vi "RSZVB Calibration Auto with Timeout.vi"(0 "VISA session":refnum<visa-resource-name>, 1 "Channel (1)":i32=1, 2 "Calibration Kit Name":string, 3 "Timeout (50000 ms)":i32=50000, 5 "error in (no error)":errorcluster {"code" format="%.0x"}, 6 "Analyzer Port 1 (1)":i32=1, 7 "Cal Unit Port 1 (1)":i32=1, 8 "Analyzer Port 2 (1)":i32=1, 9 "Cal Unit Port 2 (1)":i32=1, 10 "Analyzer Port 3 (1)":i32=1, 11 "Cal Unit Port 3 (1)":i32=1, 12 "Analyzer Port 4 (1)":i32=1, 13 "Cal Unit Port 4 (1)":i32=1) -> (14 "dup VISA session":refnum<visa-resource-name>, 19 "error out":errorcluster {"code" format="%.0x"})   [LabVIEW 2011]
doc: "This VI selects and initiates a one-port, two-port, three-port or four-port automatic calibration at arbitrary analyzer and calibration unit ports.\n\nNote(s):\n\n(1) Port numbers of the analyzer:\nFor an n-port automatic calibration (n = 1 to 4), n arbitrary (not necessarily consecutive) port numbers must be specified.\n\n(2) Port numbers of the cal unit:\nFor an n-port automatic calibration (n = 1 to 4), n arbitrary (not necessarily consecutive) port numbers must be specified. It is possible to combine arbitrary (not necessarily matching) pairs of analyzer and cal unit ports.\n \nRemote-control command(s):\n[SENSe<Ch>:]CORRection:COLLect:AUTO:PORTs '<file_name>',<analyzer_port_no>,<cal_unit_port_no>{,<analyzer_port_no>,<cal_unit_port_no>}"
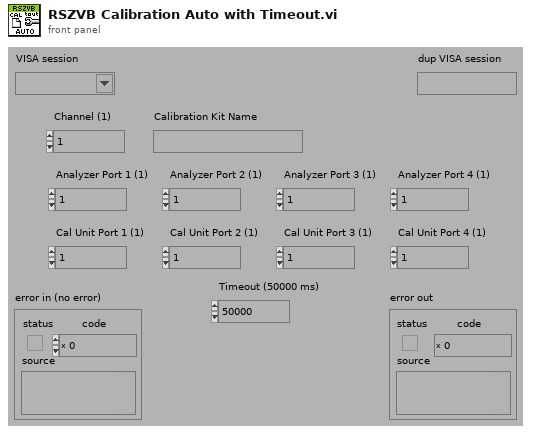
[diagram p1: front panel]
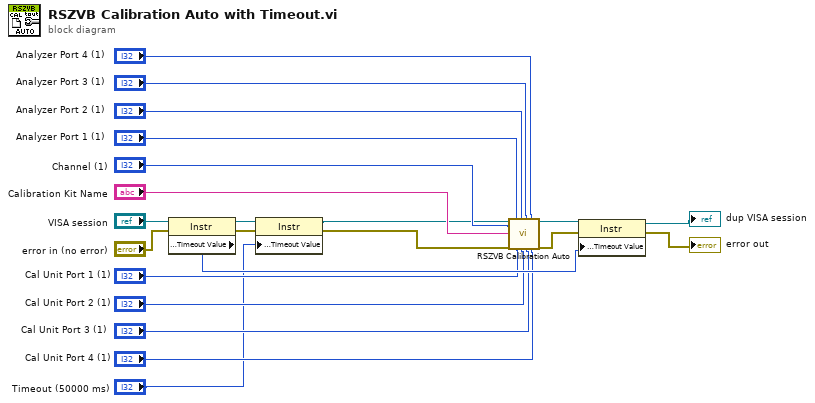
[diagram p0: block diagram]
diagram:
  n1 = property class="Instr"(reference="VISA session", error in="error in (no error)") -> (reference out=w5:refnum<visa-resource-name>, error out=w4:errorcluster, "General Settings:Timeout Value"=w20:u32)
  n2 = property class="Instr"(reference=w5, error in=w4, "General Settings:Timeout Value"="Timeout (50000 ms)") -> (reference out=w1:refnum<visa-resource-name>, error out=w2:errorcluster)
  n3 = call "RSZVB Calibration Auto.vi"("VISA session"=w1, "Channel (1)"="Channel (1)", "Calibration Kit Name"="Calibration Kit Name", "error in (no error)"=w2, "Analyzer Port 1 (1)"="Analyzer Port 1 (1)", "Cal Unit Port 1 (1)"="Cal Unit Port 1 (1)", "Analyzer Port 2 (1)"="Analyzer Port 2 (1)", "Cal Unit Port 2 (1)"="Cal Unit Port 2 (1)", "Analyzer Port 3 (1)"="Analyzer Port 3 (1)", "Cal Unit Port 3 (1)"="Cal Unit Port 3 (1)", "Analyzer Port 4 (1)"="Analyzer Port 4 (1)", "Cal Unit Port 4 (1)"="Cal Unit Port 4 (1)") -> ("dup VISA session"=w17:refnum<visa-resource-name>, "error out"=w16:errorcluster)  [unwired: 6 in]
  n4 = property class="Instr"(reference=w17, error in=w16, "General Settings:Timeout Value"=w20) -> (reference out=→"dup VISA session":refnum<visa-resource-name>, error out=→"error out":errorcluster)
